vi "NATS Publish (Polymorphic).vi"   [LabVIEW 2024, in "NATS Core.lvlib"]
doc: "Publishes a message to the NATS server. The instances of this polymorphic VI allow or disallow the inclusion of headers in a message by selecting between HPUB or PUB, respectively."
uses:
  NATS Core.lvlib
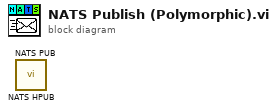
[diagram p0: block diagram]
diagram:
  n1 = call "NATS HPUB.vi"() -> ()  [unwired: 10 in, 2 out]
  n2 = call "NATS PUB.vi"() -> ()  [unwired: 10 in, 2 out]
